vi "GetText.vi"(8 "error in":errorcluster, 11 "TDMS datalogger editor node in":refnum<class "TDMS datalogger editor node.lvclass">) -> (0 "error out":errorcluster, 1 "additional text":string, 2 "text":string, 3 "TDMS datalogger editor node out":refnum<class "TDMS datalogger editor node.lvclass">, 4 "glyph":string)   [LabVIEW 2015, in "TDMS datalogger editor node.lvclass"]
uses:
  TDMS datalogger editor node.lvclass
  <vilib>/NI/DCAF/Tag Editor Core/Configuration Editor/Classes/Module editor node/module editor node.lvclass
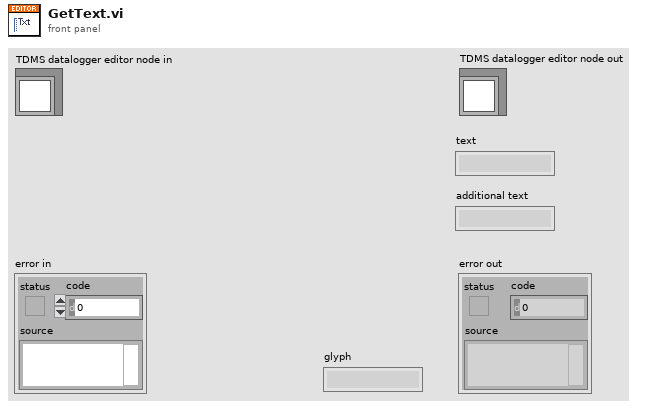
[diagram p1: front panel]
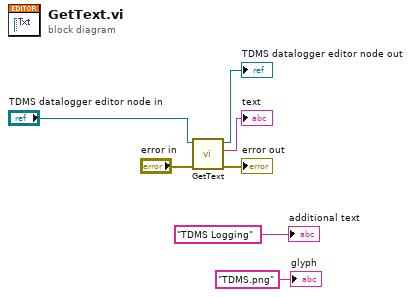
[diagram p0: block diagram]
diagram:
  n1 = call-parent "GetText.vi"("error in"="error in", "Module Editor Node in"="TDMS datalogger editor node in") -> ("error out"=→"error out":errorcluster, "text"=→"text":string, "Module Editor Node out"=→"TDMS datalogger editor node out":refnum<class "TDMS datalogger editor node.lvclass">)  [unwired: 5 in, 2 out]
  "additional text" <- "TDMS Logging" ("text")
  "glyph" <- "TDMS.png" ("glyph")
